vi "str-rip-nonchars.vi"(6 "decimate multiple whitespaces":bool, 8 "clip string (0=no clipping, pos: clip, neg: clip and stop at first non printable":i32, 11 "String_in":string) -> (3 "String_Out":string)   [LabVIEW 2014]
uses:
  <vilib>/Utility/error.llb/whitespace.ctl
panel:
  # "entferne alle nichtdruckbaren zeichen aus dem string\nzeilenumbrüche werden zu space, tab wird zu space"
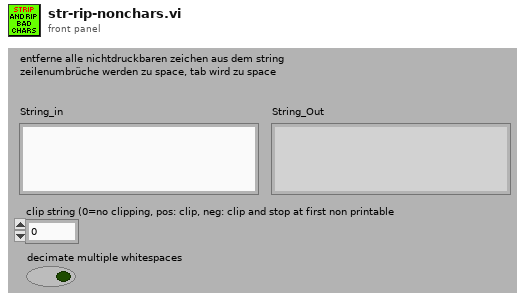
[diagram p1: front panel]
types:
  T1 = typedef "whitespace.ctl" = u16
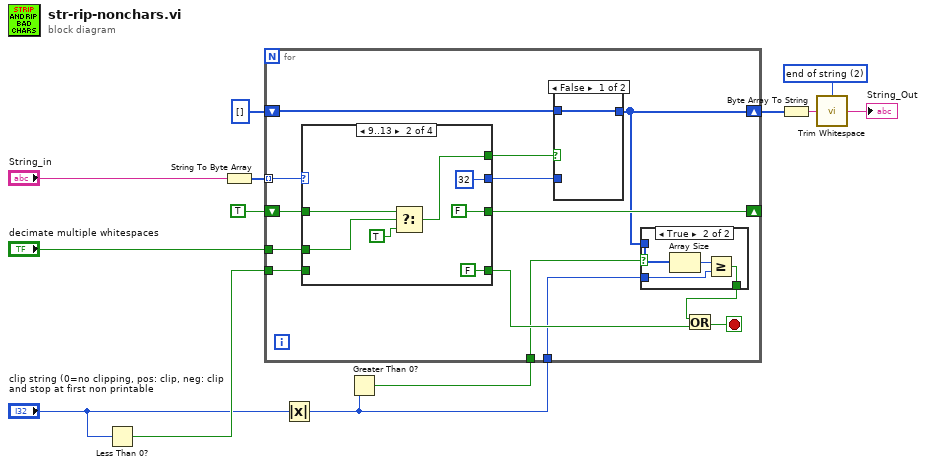
[diagram p0: block diagram]
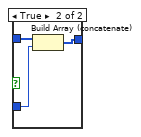
[diagram p3: hidden frame]
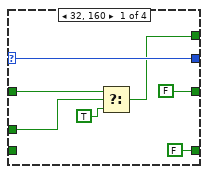
[diagram p4: hidden frame]
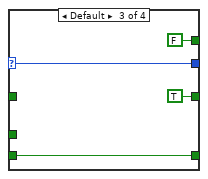
[diagram p5: hidden frame]
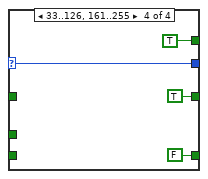
[diagram p6: hidden frame]
diagram:
  w1 = T1 2 items=["both", "start of string", "end of string"] ("location (both)")
  n1 = Less Than 0?(x="clip string (0=no clipping, pos: clip, neg: clip and stop at first non printable") -> (x < 0?=w10:bool)
  n2 = String To Byte Array(string="String_in") -> (unsigned byte array=w13:u8[])
  n3 = Absolute Value(x="clip string (0=no clipping, pos: clip, neg: clip and stop at first non printable") -> (abs(x)=w5:i32)
  n4 = Greater Than 0?(x=w5) -> (x > 0?=w4:bool)
  n5 = for {
    tunnel: w13 -> [w27] mode=indexing
    shift-right: [w14] -> w11
    shift-left: u8[] [] -> [w26]
    shift-right: [w20] -> _
    shift-left: TRUE -> [w24]
    tunnel: w10 -> [w23]
    tunnel: "decimate multiple whitespaces" -> [w22]
    tunnel: w5 -> [w18]
    tunnel: w4 -> [w17]
    stop <- w15 stop-if-true
    n6 = case shown="9..13" w27 {
      selector: w27 -> [w43 _ w52 w58]
      tunnel: [w43 u8 32 w52 w58] -> w25
      tunnel: w24 -> [w38 w46 _ _]
      tunnel: [w39 w47 FALSE TRUE] -> w21
      tunnel: w23 -> [_ _ w53 _]
      tunnel: [FALSE FALSE w53 FALSE] -> w19
      tunnel: w22 -> [w41 w49 _ _]
      tunnel: [FALSE FALSE TRUE TRUE] -> w20
      frame 32, 160 {
        n7 = Select(t=w38, s=w41, f=TRUE) -> (s? t:f=w39:bool)
      }
      frame 9..13 {
        n8 = Select(t=w46, s=w49, f=TRUE) -> (s? t:f=w47:bool)
      }
      frame Default {
      }
      frame 33..126, 161..255 {
      }
    }
    n9 = case shown="False" w21 {
      tunnel: [w33 w36] -> w14
      tunnel: w26 -> [w33 w35]
      tunnel: w25 -> [_ w34]
      frame False {
      }
      frame True {
        n10 = Build Array (concatenate)(w35, w34) -> (w36:u8[])
      }
    }
    n11 = case shown="True" w17 {
      selector: w17 -> [w28 _]
      tunnel: w14 -> [_ w32]
      tunnel: w18 -> [_ w30]
      tunnel: [w28 w29] -> w16
      frame False {
      }
      frame True {
        n12 = Array Size(array=w32) -> (size(s)=w31:i32)
        n13 = Greater Or Equal?(x=w31, y=w30) -> (x >= y?=w29:bool)
      }
    }
    n14 = Or(x=w16, y=w19) -> (x .or. y?=w15:bool)
  }
  n15 = Byte Array To String(unsigned byte array=w11) -> (string=w3:string)
  n16 = call <vilib>:"Trim Whitespace.vi"("string"=w3, "location (both)"=w1) -> ("trimmed string"=→"String_Out":string)
